vi "Encoder Math.vi"(2 "Encoder A_old":bool, 3 "Encoder B_old":bool, 4 "Encoder A_new":bool, 5 "Encoder B_new":bool) -> (0 "The Encoder Changed":bool, 1 "Change in Encoder Value":i32)   [LabVIEW 2009]
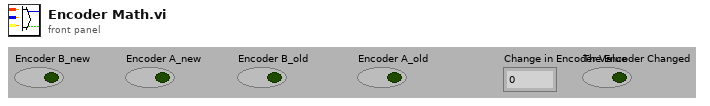
[diagram p1: front panel]
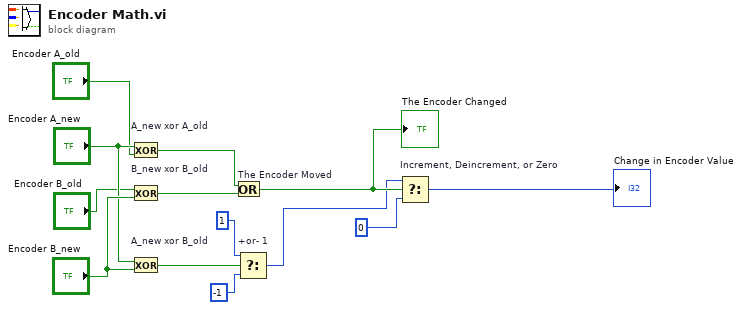
[diagram p0: block diagram]
diagram:
  n1 = Exclusive Or "A_new xor A_old"(1:"Encoder A_old", 2:"Encoder A_new") -> (0:w2:bool)
  n2 = Exclusive Or "B_new xor B_old"(1:"Encoder B_new", 2:"Encoder B_old") -> (0:w3:bool)
  n3 = Exclusive Or "A_new xor B_old"(1:"Encoder B_new", 2:"Encoder A_new") -> (0:w9:bool)
  n4 = Or "The Encoder Moved"(x=w2, y=w3) -> (x .or. y?=w12:bool)
  "The Encoder Changed" <- w12
  n5 = Select "+or- 1"(t=1 ("16 bit"), s=w9, f=-1 ("16 bit")) -> (s? t:f=w10:i32)
  n6 = Select "Increment, Deincrement, or Zero"(t=w10, s=w12, f=0) -> (s? t:f=→"Change in Encoder Value":i32)
